vi "TestLoadVi.vi"() -> ()   [LabVIEW 2009, in "MoAgSy_TEST.lvlib"]
uses:
  MoAgSy_TEST/MoAgSy_TEST.lvlib
  MoAgSy_Factory/MoAgSy_Factory.lvclass
  MoAgSy_AgentBase/MoAgSy_AgentBase.lvclass
  HGF_BaseClasses/HGF_Factory/HGF_Factory.lvclass
panel:
  out "Control Value:Get All":cluster{"Name":string, "Variant Data":variant}[](array[cluster])
  out "error out":errorcluster
  out "Agents":string[](array[string])
  out "Factories":path[](array[path])
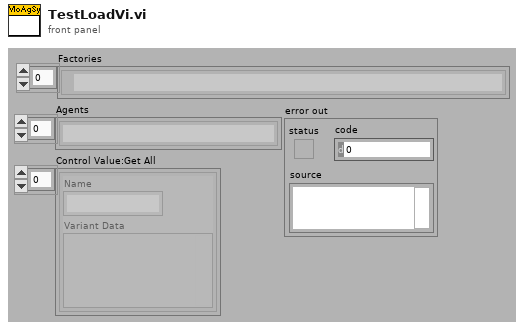
[diagram p1: front panel]
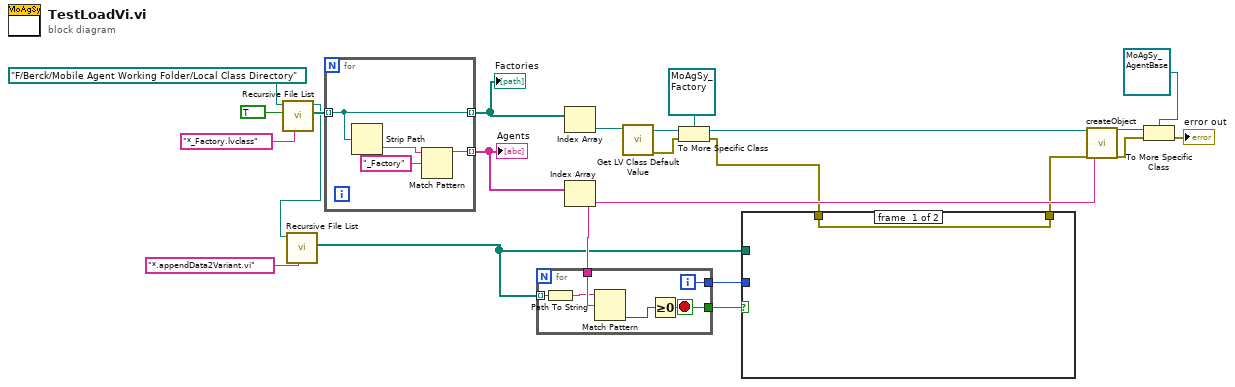
[diagram p0: block diagram]
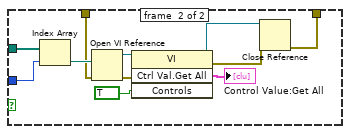
[diagram p2: hidden frame]
diagram:
  n1 = call <vilib>:"Recursive File List.vi"("pattern"="*_Factory.lvclass", "Treat LLBs as Folders?"=TRUE, "Folder Path"=path "F:/Berck/Mobile Agent Working Folder/Local Class Directory") -> ("All Files in Dir"=w20:path[], "dup Folder Path"=w9:path)  [unwired: 4 in, 3 out]
  n2 = call <vilib>:"Recursive File List.vi"("pattern"="*.appendData2Variant.vi", "Folder Path"=w9) -> ("All Files in Dir"=w6:path[])  [unwired: 5 in, 4 out]
  n3 = for {
    tunnel: w20 -> [w27] mode=indexing
    tunnel: [w27] -> w19 mode=indexing
    tunnel: [w26] -> w13 mode=indexing
    n4 = Strip Path(path=w27) -> (name=w25:string)  [unwired: 1 out]
    n5 = Match Pattern(string=w25, regular expression="_Factory") -> (before substring=w26:string)  [unwired: 1 in, 3 out]
  }
  "Factories" <- w19
  "Agents" <- w13
  n6 = Index Array(array=w19) -> (element=w18:path)  [unwired: 1 in]
  n7 = Index Array(array=w13) -> (element=w7:string)  [unwired: 1 in]
  n8 = for {
    tunnel: w7 -> [w33]
    tunnel: [w31] -> w5
    tunnel: w6 -> [w30] mode=indexing
    tunnel: [w28] -> w4
    i -> [w28]
    stop <- w31 stop-if-true
    n9 = Path To String(path=w30) -> (string=w29:string)
    n10 = Match Pattern(string=w29, regular expression=w33) -> (offset past match=w32:i32)  [unwired: 1 in, 3 out]
    n11 = Greater Or Equal To 0?(x=w32) -> (x >= 0?=w31:bool)
  }
  n12 = call <vilib>:"Get LV Class Default Value.vi"("class path"=w18) -> ("error out"=w16:errorcluster, "object"=w17:refnum<class>)  [unwired: 9 in]
  n13 = To More Specific Class(target class=refnum<class "MoAgSy_Factory.lvclass"> refnum ("MoAgSy_Base.lvlib:MoAgSy_Factory.lvclass"), reference=w17, error in=w16) -> (specific class reference=w14:refnum<class "MoAgSy_Factory.lvclass">, error out=w3:errorcluster)
  n14 = case shown="True" w5 {
    tunnel: w6 -> [_ w45]
    tunnel: w4 -> [_ w44]
    tunnel: w3 -> [w34 w38]
    tunnel: [w34 w37] -> w2
    frame #0 {
    }
    frame #1 {
      n15 = Index Array(array=w45, index=w44) -> (element=w43:path)
      n16 = Open VI Reference(vi path=w43, error in (no error)=w38) -> (vi reference=w41:refnum<vi>, error out=w42:errorcluster)  [unwired: 4 in]
      n17 = invoke class="VI" method="Ctrl Val.Get All"(reference=w41, error in=w42, "Controls"=TRUE) -> (reference out=w40:refnum<vi>, error out=w39:errorcluster, "Get All Control Values Variant"=→"Control Value:Get All":cluster{"Name":string, "Variant Data":variant}[])  [unwired: 1 in, 1 out]
      n18 = Close Reference(reference=w40, error in (no error)=w39) -> (error out=w37:errorcluster)
    }
  }
  n19 = call "createObject.vi"("HGF_Factory"=w14, "error in (no error)"=w2, "className"=w7) -> ("HGF_Object"=w11:refnum<class "HGF_Factory.lvclass">, "error out"=w12:errorcluster)  [unwired: 14 in, 1 out]
  n20 = To More Specific Class(target class=refnum<class "MoAgSy_AgentBase.lvclass"> refnum ("MoAgSy_Base.lvlib:MoAgSy_AgentBase.lvclass"), reference=w11, error in=w12) -> (error out=→"error out":errorcluster)  [unwired: 1 out]
